vi "load_cv_data.vi"(7 "matched set":set{cluster{"CLZ id":i32, "CV id":i32}}(c389), 8 "error in (no error)":errorcluster, 10 "binary folder":path, 11 "Volumes in":refnum<class "CV Comics.lvclass">) -> (0 "error out":errorcluster, 2 "cv issue map":map{i32, T1}(c390), 3 "Volumes out":refnum<class "CV Comics.lvclass">)   [LabVIEW 2024, in "CLZ_to_ComicVine.lvlib" / "CV Comics.lvclass"]
uses:
  CV Comics.lvclass
  comic_manager/manager_daemon/type_defs/IssueData--clustrer.ctl
  comic_manager/manager_daemon/type_defs/VolumeData--cluster.ctl
  CV_Shared_Library/volume.type--enum.ctl
  typedefs/volume--cluster.ctl
  CV Comics.lvclass/CV Comics.ctl
  CV_Shared_Library/CV_Shared_Library.lvlib
  comic_manager/manager_daemon/manager_daemon.lvclass
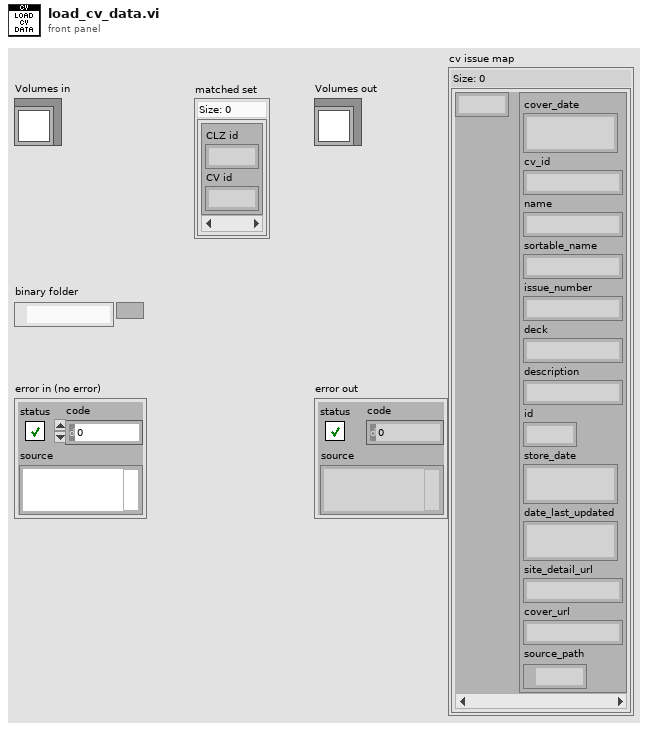
[diagram p1: front panel]
types:
  T1 = typedef "manager_daemon.lvclass/IssueData--clustrer.ctl" = cluster{"cover_date":timestamp, "cv_id":string, "name":string, "sortable_name":string, "issue_number":string, "deck":string, "description":string, "id":i32, "store_date":timestamp, "date_last_updated":timestamp, "site_detail_url":string, "cover_url":string, "source_path":path}
  T2 = typedef "CLZ_to_ComicVine.lvlib/CV Comics.lvclass/volume--cluster.ctl" = cluster{"id":i32, "name":string, "issue set":set{string}, "matched":bool}
  T3 = typedef "manager_daemon.lvclass/VolumeData--cluster.ctl" = cluster{"name":string, "sortable_name":string, "aliases":string[], "description":string, "site_detail_url":string, "count_of_issues":i32, "start_year":i32, "publisher_id":i32, "issue_ids":i32[], "date_last_updated":timestamp, "volume":i32, "cv_id":string, "volume type":T4, "source_path":path}
  T4 = typedef "CV_Shared_Library.lvlib/volume.type--enum.ctl" = enum16{"Ongoing", "Limited Series", "Annual", "One Shot", "Reprint/Document", "Star Comics", "Epic Comics"}
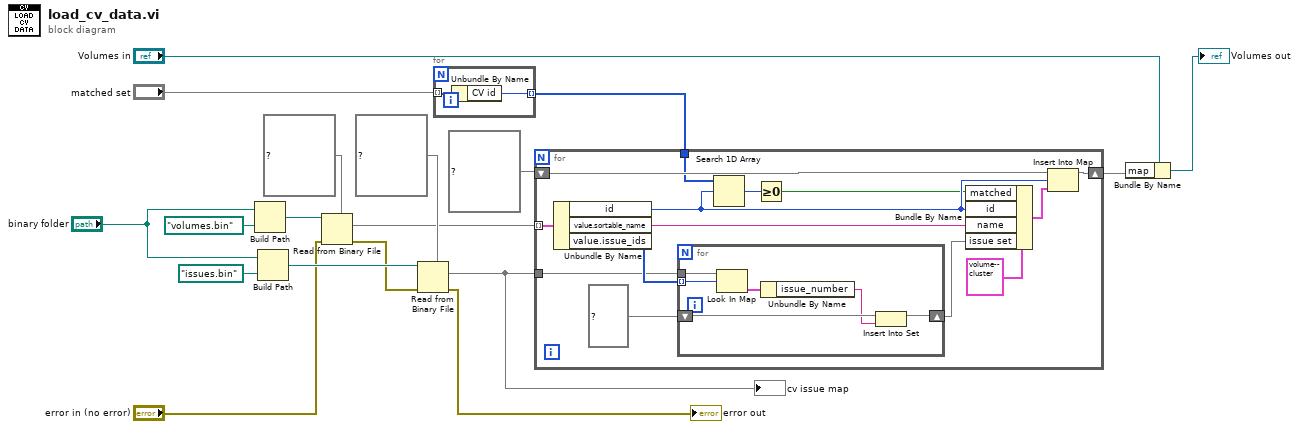
[diagram p0: block diagram]
diagram:
  n1 = Build Path(base path="binary folder", name or relative path=path "volumes.bin") -> (appended path=w14:path)
  n2 = Build Path(base path="binary folder", name or relative path=path "issues.bin") -> (appended path=w12:path)
  n3 = Read from Binary File(5:map{i32, T3} {} ("volume map"), 8:"error in (no error)", 11:w14) -> (0:w10:errorcluster, 2:w8:map{i32, T3})  [unwired: 3 in, 2 out]
  n4 = Read from Binary File(5:map{i32, T1} {} ("issue map"), 8:w10, 11:w12) -> (0:→"error out":errorcluster, 2:w1:map{i32, T1})  [unwired: 3 in, 2 out]
  "cv issue map" <- w1
  n5 = for {
    tunnel: "matched set" -> [w20] mode=indexing
    tunnel: [w19] -> w2 mode=indexing
    n6 = Unbundle By Name(w20) -> ("CV id"=w19:i32)
  }
  n7 = for {
    tunnel: w8 -> [w34] mode=indexing
    tunnel: w1 -> [w32]
    shift-right: [w26] -> w5
    shift-left: map{i32, T2} {} ("map") -> [w27]
    tunnel: w2 -> [w24]
    n8 = Unbundle By Name(w34) -> ("id"=w23:i32, "value.sortable_name"=w29:string, "value.issue_ids"=w33:i32[])
    n9 = for {
      tunnel: w33 -> [w39] mode=indexing
      tunnel: w32 -> [w40]
      shift-right: [w37] -> w28
      shift-left: set{string} {} ("issue set") -> [w36]
      n10 = Look In Map(map=w40, key=w39) -> (value=w38:T1)  [unwired: 1 in, 1 out]
      n11 = Unbundle By Name(w38) -> ("issue_number"=w35:string)
      n12 = Insert Into Set(10:w35, 11:w36) -> (3:w37:set{string})  [unwired: 1 out]
    }
    n13 = Search 1D Array(1D array=w24, element=w23) -> (index of element=w22:i32)  [unwired: 1 in]
    n14 = Greater Or Equal To 0?(x=w22) -> (x >= 0?=w21:bool)
    n15 = Bundle By Name(cluster=T2 {"id"=0, "name"="", "issue set"={}, "matched"=FALSE} ("volume"), "matched"=w21, "id"=w23, "name"=w29, "issue set"=w28) -> (w25:T2)
    n16 = Insert Into Map(map in=w27, key=w23, value=w25) -> (map out=w26:map{i32, T2})  [unwired: 2 out]
  }
  n17 = Bundle By Name(cluster="Volumes in", "map"=w5) -> (→"Volumes out":refnum<class "CV Comics.lvclass">)
